vi "Sanitize.vi"(8 "error in (no error)":errorcluster, 11 "RawTag":string) -> (0 "error out":errorcluster, 3 "CleanTag":string)   [LabVIEW 2026, in "Lumberjack.lvlib"]
doc: "Pure tag sanitization. Convert a raw string into a single valid hierarchy node by replacing every space and dot with an underscore, so a VI-derived name does not read as a false dot-separated hierarchy (SRS-LMBR-013). Trims leading and trailing whitespace first. No state, no I/O; deterministic."
uses:
  Lumberjack.lvlib
  <vilib>/Utility/error.llb/Trim Whitespace (string).vi
  <vilib>/Utility/error.llb/Trim Whitespace One-Sided.vi
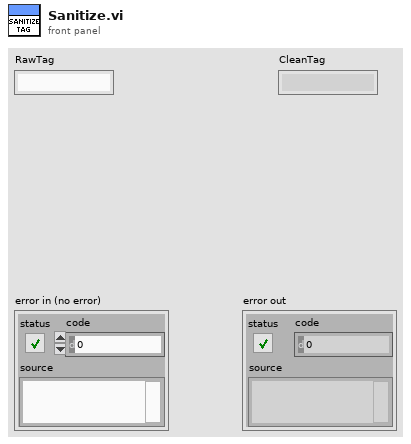
[diagram p1: front panel]
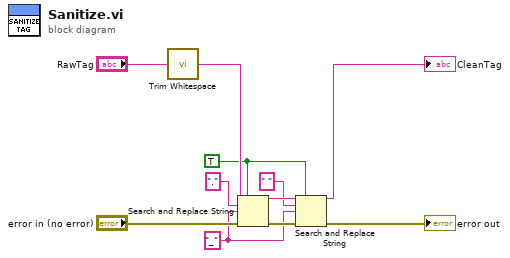
[diagram p0: block diagram]
diagram:
  w1 = TRUE ("replace all? (F)")
  w5 = "_" ("replace string (\"\")")
  n1 = call-poly <vilib>:"Trim Whitespace.vi"("string"="RawTag") -> ("trimmed string"=w3:string)  [unwired: 1 in]
  n2 = Search and Replace String(replace all?=w1, input string=w3, search string=".", replace string=w5, error in="error in (no error)") -> (result string=w6:string, error out=w8:errorcluster)  [unwired: 3 in, 2 out]
  n3 = Search and Replace String(replace all?=w1, input string=w6, search string=" ", replace string=w5, error in=w8) -> (result string=→"CleanTag":string, error out=→"error out":errorcluster)  [unwired: 3 in, 2 out]
